vi "SelectHandle.vi"(8 "error in (no error)":errorcluster, 11 "SyncPlugin":refnum<class "SyncPluginBase.lvclass">) -> (0 "error out":errorcluster, 3 "SyncPlugin":refnum<class "SyncPluginBase.lvclass">)   [LabVIEW 2014]
uses:
  <userlib>/NIST/BaseClasses/Object_class/BaseObject.lvclass
  SyncPluginBase.lvclass
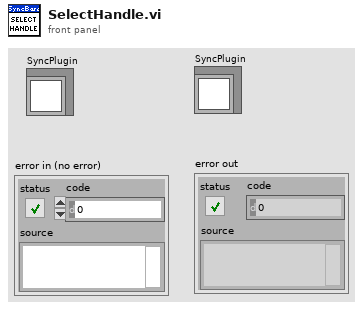
[diagram p1: front panel]
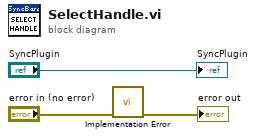
[diagram p0: block diagram]
diagram:
  n1 = call <userlib>:"Implementation Error.vi"("error in (no error)"="error in (no error)") -> ("error out"=→"error out":errorcluster)  [unwired: 10 in]
  "SyncPlugin" <- "SyncPlugin"
